vi "Elevator Offset AutoMatic.vi"() -> ()   [LabVIEW 2014]
uses:
  <vilib>/Rock Robotics/WPI/Joystick/WPI_JoystickGetSetRefNum.vi
panel:
  in  "Time Step(ms)":u32=10
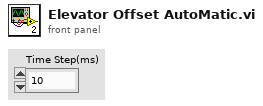
[diagram p1: front panel]
types:
  T1 = typedef "WPI_JoystickDevRef.ctl" = cluster{"Device":T2}
  T2 = typedef "WPI_JoystickDeviceEnum.ctl" = enum16{"USB 0", "USB 1", "USB 2", "USB 3", "USB 4", "USB 5"}
  T3 = typedef "WPI_MotorControlDeviceRef.ctl" = cluster{"DeviceStatus":errorcluster, "Type":T4, "PWM":cluster{"Controller":T5, "PWM Channel":T6, "DeadBand":T7}, "CAN":cluster{"Device Number":u8, "Control Mode":T8, "Semaphore":T9, "Max Vout":dbl, "TalonSRX Control Mode":T10}, "Invert":bool, "TransformRef":T11, "InvTransformRef":T11}
  T4 = typedef "WPI_MotorControlType.ctl" = enum16{"PWM", "CAN", "CANTalonSRX"}
  T5 = typedef "FPGA_TypedefDigitalModule.ctl" = enum16{"Controller 1"}
  T6 = typedef "FPGA_DIOPWMChannel.ctl" = enum8{"PWM 0", "PWM 1", "PWM 2", "PWM 3", "PWM 4", "PWM 5", "PWM 6", "PWM 7", "PWM 8", "PWM 9", "PWM MXP 0", "PWM MXP 1", "PWM MXP 2", "PWM MXP 3", "PWM MXP 4", "PWM MXP 5", "PWM MXP 6", "PWM MXP 7", "PWM MXP 8", "PWM MXP 9", "Invalid"}
  T7 = typedef "WPI_PWMDeadband.ctl" = cluster{"Name":string, "maxPositivePwm":i32, "minPositivePwm":i32, "centerPwm":i32, "maxNegativePwm":i32, "minNegativePwm":i32, "angularRange":u16}
  T8 = typedef "WPI_CANJaguar_ControlMode.ctl" = enum8{"Percent VBus", "Current", "Speed", "Position", "Voltage"}
  T9 = typedef "Semaphore RefNum" = refnum<k1>
  T10 = typedef "WPI_CANTalonSRX_APIControlMode.ctl" = enum8{"Percent VBus", "Speed", "Position", "Slave", "Unchanged / Invalid"}
  T11 = typedef "WPI_PWMTransform_ConPane.ctl" = refnum<vi>
  T12 = typedef "WPI_CANTalonSRX_GlobalStatus.ctl" = cluster{"Applied Throttle":dbl, "Module Enabled":bool, "CAN Error":errorcluster, "Closed Loop Error":dbl, "Forward Limit Switch Closed":bool, "Reverse Limit Switch Closed":bool, "Sensor Position":dbl, "Sensor Velocity":dbl, "Current":dbl, "Sticky Fault - Over Temp":bool, "Sticky Fault - Under Voltage":bool, "Sticky Fault - Forward Limit":bool, "Sticky Fault - Reverse Limit":bool, "Sticky Fault - Forward Soft Limit":bool, "Sticky Fault - Reverse Soft Limit":bool, "Brake is Enabled":bool, "Encoder Position":dbl, "Encoder Velocity":dbl, "Encoder Index Count":dbl, "Encoder A Pin State":bool, "Encoder B Pin State":bool, "Encoder Index Pin State":bool, "Analog In":dbl, "Analog In Velocity":dbl, "Temperature (C)":dbl, "Battery Voltage":dbl}
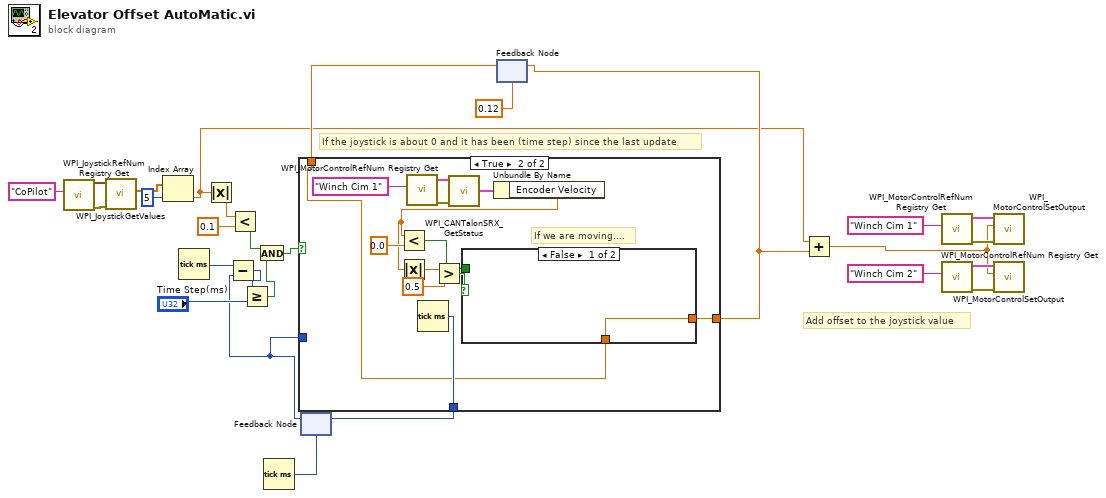
[diagram p0: block diagram]
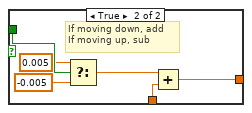
[diagram p3: hidden frame]
diagram:
  # "Add offset to the joystick value"
  # "If the joystick is about 0 and it has been (time step) since the last update"
  n1 = call <vilib>:"WPI_JoystickRefNum Registry Get.vi"("refnum name"="CoPilot") -> ("error out"=w15:errorcluster, "JoystickDevRef"=w16:T1)  [unwired: 9 in]
  n2 = call <vilib>:"WPI_JoystickGetValues.vi"("error in (no error)"=w15, "JoystickDevRef"=w16) -> ("Axes"=w14:dbl[])  [unwired: 5 in, 4 out]
  n3 = Index Array(array=w14, index=5) -> (element=w2:dbl)
  n4 = Tick Count (ms)() -> (millisecond timer value=w19:u32)
  n5 = Absolute Value(x=w2) -> (abs(x)=w8:dbl)
  n6 = Less?(x=w8, y=0.1) -> (x < y?=w6:bool)
  n7 = Tick Count (ms)() -> (millisecond timer value=w20:u32)
  n8 = feedback #1(w20) -> (w9:u32)
  n9 = Subtract(x=w19, y=w9) -> (x-y=w18:u32)
  n10 = Greater Or Equal?(x=w18, y="Time Step(ms)") -> (x >= y?=w11:bool)
  n11 = And(x=w6, y=w11) -> (x .and. y?=w12:bool)
  n12 = feedback #2(0.12) -> (w4:dbl)
  n13 = case shown="True" w12 {
    tunnel: [w29 w38] -> w10
    tunnel: w9 -> [w29 _]
    tunnel: w4 -> [w28 w31]
    tunnel: [w28 w30] -> w3
    frame False {
    }
    frame True {
      # "If we are moving...."
      n14 = call <vilib>:"WPI_MotorControlRefNum Registry Get.vi"("refnum name"="Winch Cim 1") -> ("error out"=w40:errorcluster, "MotorControlDevRef"=w41:T3)  [unwired: 9 in]
      n15 = Tick Count (ms)() -> (millisecond timer value=w38:u32)
      n16 = call <vilib>:"WPI_CANTalonSRX_GetStatus.vi"("error in (no error)"=w40, "CAN Talon SRX Ref"=w41) -> ("Talon SRX Status"=w39:T12)  [unwired: 7 in, 2 out]
      n17 = Unbundle By Name(w39) -> ("Encoder Velocity"=w36:dbl)
      n18 = Less?(x=w36, y=0.0) -> (x < y?=w32:bool)
      n19 = Absolute Value(x=w36) -> (abs(x)=w35:dbl)
      n20 = Greater?(x=w35, y=0.5) -> (0:w33:bool)
      n21 = case shown="False" w33 {
        tunnel: w32 -> [_ w49]
        tunnel: w31 -> [w43 w45]
        tunnel: [w43 w44] -> w30
        frame False {
        }
        frame True {
          # "If moving down, add\nIf moving up, sub"
          n22 = Select(t=0.005, s=w49, f=-0.005) -> (s? t:f=w46:dbl)
          n23 = Add(x=w46, y=w45) -> (x+y=w44:dbl)
        }
      }
    }
  }
  n24 = feedback-in #1(w10) -> ()
  n25 = feedback-in #2(w3) -> ()
  n26 = Add(x=w2, y=w3) -> (x+y=w1:dbl)
  n27 = call <vilib>:"WPI_MotorControlRefNum Registry Get.vi"("refnum name"="Winch Cim 1") -> ("error out"=w26:errorcluster, "MotorControlDevRef"=w25:T3)  [unwired: 9 in]
  n28 = call <vilib>:"WPI_MotorControlRefNum Registry Get.vi"("refnum name"="Winch Cim 2") -> ("error out"=w23:errorcluster, "MotorControlDevRef"=w22:T3)  [unwired: 9 in]
  n29 = call <vilib>:"WPI_MotorControlSetOutput.vi"("error in (no error)"=w26, "Output"=w1, "MotorControlDevRef"=w25) -> ()  [unwired: 6 in, 3 out]
  n30 = call <vilib>:"WPI_MotorControlSetOutput.vi"("error in (no error)"=w23, "Output"=w1, "MotorControlDevRef"=w22) -> ()  [unwired: 6 in, 3 out]
